vi "Setup.vi"(8 "error in (no error)":errorcluster, 10 "Libray Path":path, 11 "TestRunner in":refnum<class "TestRunner.lvclass">) -> (0 "error out":errorcluster, 3 "TestRunner out":refnum<class "TestRunner.lvclass">)   [LabVIEW 2019, in "TestRunner.lvlib" / "TestRunner.lvclass"]
uses:
  TestRunner.lvclass
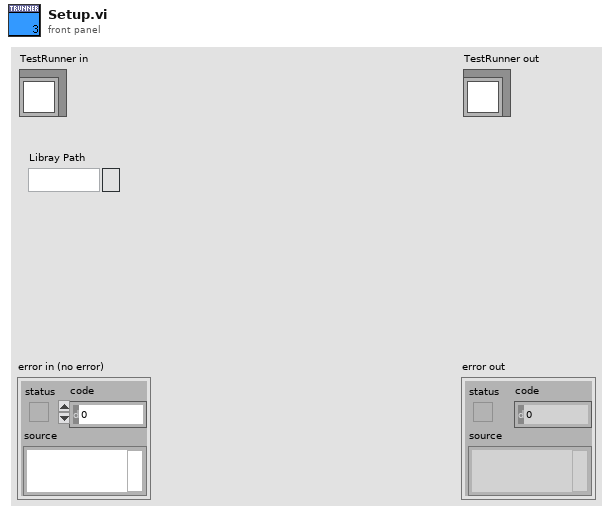
[diagram p1: front panel]
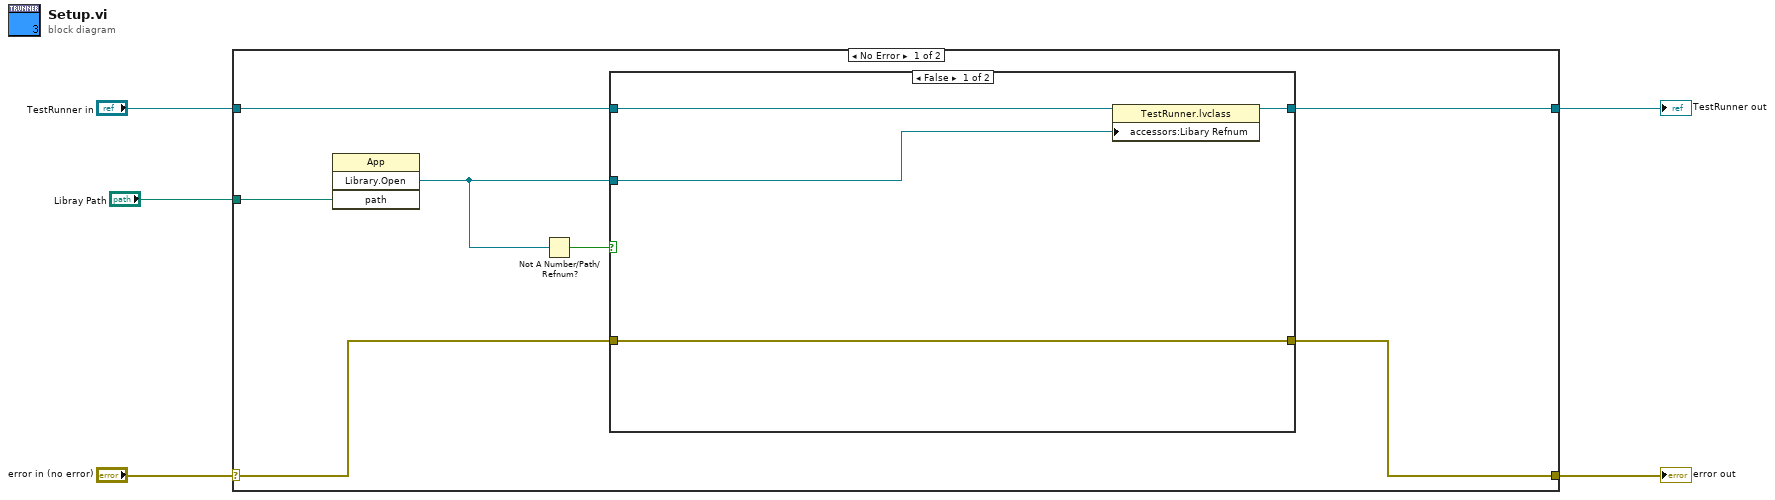
[diagram p0: block diagram]
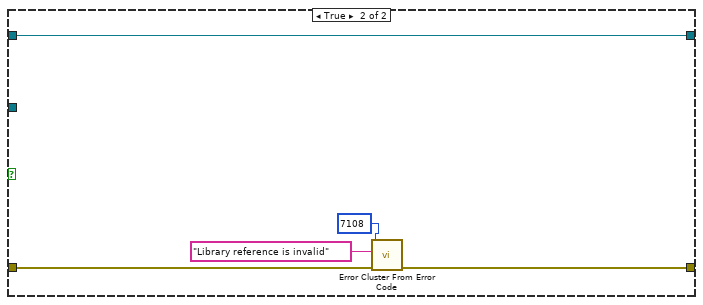
[diagram p2: hidden frame]
diagram:
  n1 = case shown="No Error" "error in (no error)" {
    selector: "error in (no error)" -> [w9 w23]
    tunnel: [w8 w23] -> w4
    tunnel: [w11 w22] -> w2
    tunnel: "TestRunner in" -> [w12 w22]
    tunnel: "Libray Path" -> [w7 _]
    frame No Error {
      n2 = invoke class="App" method="Library.Open"("path"=w7) -> ("Open Library"=w10:refnum<vi>)  [unwired: 3 in, 3 out]
      n3 = Not A Number/Path/Refnum?(number/path/refnum=w10) -> (NaN/Path/Refnum?=w6:bool)
      n4 = case shown="False" w6 {
        tunnel: w12 -> [w16 w21]
        tunnel: [w14 w21] -> w11
        tunnel: w10 -> [w13 _]
        tunnel: w9 -> [w15 w18]
        tunnel: [w15 w17] -> w8
        frame False {
          n5 = property class="TestRunner.lvclass"(reference=w16, "accessors:Libary Refnum"=w13) -> (reference out=w14:refnum<class "TestRunner.lvclass">)  [unwired: 1 in, 1 out]
        }
        frame True {
          n6 = call <vilib>:"Error Cluster From Error Code.vi"("error in (no error)"=w18, "error message (\"\")"="Library reference is invalid" ("error message (\"\")"), "error code (0)"=7108) -> ("error out"=w17:errorcluster)  [unwired: 6 in]
        }
      }
    }
    frame Error {
    }
  }
  "error out" <- w4
  "TestRunner out" <- w2
